vi "Intersect.vi"(10 "before_sweep_table":dbl[](array[numeric]), 11 "sweep_table":dbl[](array[numeric])) -> (3 "before_sweep_table out":dbl[](array[numeric]))   [LabVIEW 2017]
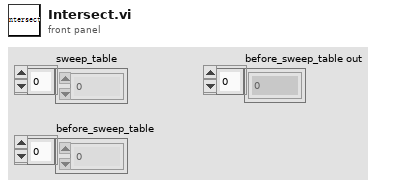
[diagram p1: front panel]
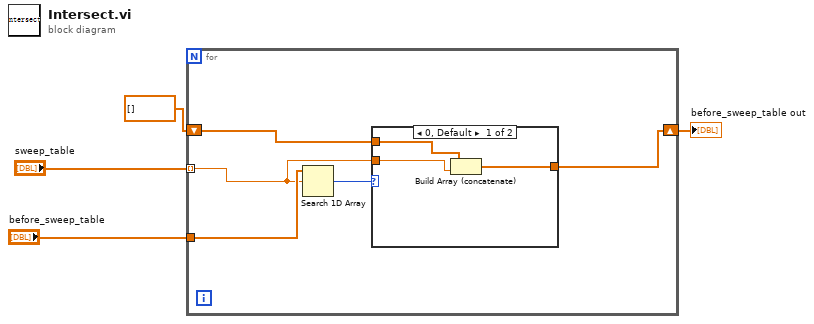
[diagram p0: block diagram]
diagram:
  n1 = for {
    tunnel: "sweep_table" -> [w7] mode=indexing
    tunnel: "before_sweep_table" -> [w8]
    shift-right: [w5] -> w4
    shift-left: dbl[] [] ("TSL_OSUport") -> [w6]
    n2 = Search 1D Array(1D array=w8, element=w7) -> (index of element=w9:i32)  [unwired: 1 in]
    n3 = case shown="0, Default" w9 {
      tunnel: w7 -> [w12 _]
      tunnel: w6 -> [w11 w13]
      tunnel: [w10 w13] -> w5
      frame 0, Default {
        n4 = Build Array (concatenate)(w11, w12) -> (w10:dbl[])
      }
      frame -1 {
      }
    }
  }
  "before_sweep_table out" <- w4
